vi "LCP Set Flow Unit.vi"(7 "Prefix":T3=-3 items=["UNIT"=0, "DECI"=-1, "CENTI"=-2, "MILLI"=-3, "MICRO"=-6], 8 "error in (no error)":errorcluster caption="Fehler (Eingang, kein Fehler)", 9 "TimeUnit":T1=60 items=["PER_SECOND"=1, "PER_MINUTE"=60, "PER_HOUR"=3600], 10 "VolumeUnit":T2 items=["LITRES"=68], 11 "Pump Handle":i64) -> (0 "error out":errorcluster caption="Fehler (Ausgang)")   [LabVIEW 2021, in "labbCAN_Pump_API.lvlib"]
doc: "LCP_Func long LCP_CALL LCP_SetFlowUnit(dev_hdl hPump,\n int Prefix,\n int VolumeUnit,\n int TimeUnit);"
uses:
  labbCAN_Pump_API.lvlib
  labbCAN_Bus_API/SiUnitPrefix.ctl
  VolumeUnits.ctl
  labbCAN_Bus_API/TimeUnits.ctl
  labbCAN_Pump_API.dll
  labbCAN_Bus_API/labbCAN_Bus_API.lvlib
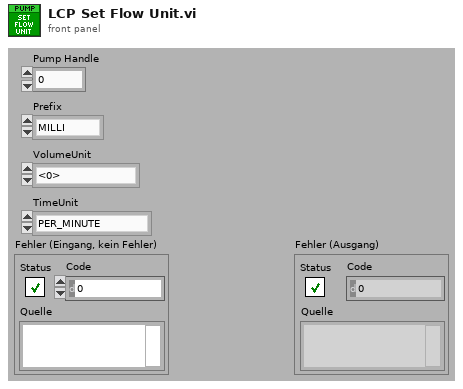
[diagram p1: front panel]
types:
  T1 = typedef "labbCAN_Bus_API.lvlib/TimeUnits.ctl" = i32
  T2 = typedef "labbCAN_Pump_API.lvlib/VolumeUnits.ctl" = i32
  T3 = typedef "labbCAN_Bus_API.lvlib/SiUnitPrefix.ctl" = i32
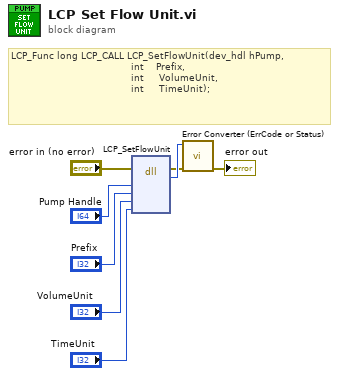
[diagram p0: block diagram]
diagram:
  # "LCP_Func long LCP_CALL LCP_SetFlowUnit(dev_hdl hPump,\n                                        int    Prefix,\n                                        int     VolumeUnit,\n                                        int     TimeUnit);"
  n1 = dll-call lib="C:/Users/olaja/AppData/Local/CETONI_SDK/labbCAN_Pump_API.*" fn="LCP_SetFlowUnit"(error in="error in (no error)", "hPump"="Pump Handle", "Prefix"="Prefix", "VolumeUnit"="VolumeUnit", "TimeUnit"="TimeUnit") -> (error out=w2:errorcluster, "Rückgabetyp"=w3:i32)  [unwired: 6 in, 1 out]
  n2 = call "Error Converter (ErrCode or Status).vi"("error in (no error)"=w2, "error code"=w3) -> ("error out"=→"error out":errorcluster)  [unwired: 9 in]
